vi "FlatToRichni_xnet_can_bm_api_ConnectSettings.vi"(5 "OutputClusterType":T1, 11 "InputCluster":T5) -> (3 "OutputCluster":T1)   [LabVIEW 2025, in "xnet_can_bus_monitor_api_client.lvlib"]
uses:
  ni_xnet_can_bm_api_ConnectSettings_Flat.ctl
  ni_xnet_can_bm_api_CanMode.ctl
  ni_xnet_can_bm_api_Termination.ctl
  ni_xnet_can_bm_api_FdIsoMode.ctl
  ni_xnet_can_bm_api_ConnectSettings.ctl
  xnet_can_bus_monitor_api_client.lvlib
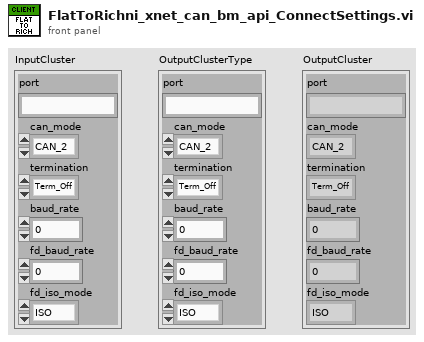
[diagram p1: front panel]
types:
  T1 = typedef "xnet_can_bus_monitor_api_client.lvlib/ni_xnet_can_bm_api_ConnectSettings.ctl" = cluster{"port":string, "can_mode":T2, "termination":T3, "baud_rate":u64, "fd_baud_rate":u64, "fd_iso_mode":T4}
  T2 = typedef "xnet_can_bus_monitor_api_client.lvlib/ni_xnet_can_bm_api_CanMode.ctl" = enum32{"CAN_2", "CAN_FD", "CAN_FD_BRS"}
  T3 = typedef "xnet_can_bus_monitor_api_client.lvlib/ni_xnet_can_bm_api_Termination.ctl" = enum32{"Term_Off", "Term_On"}
  T4 = typedef "xnet_can_bus_monitor_api_client.lvlib/ni_xnet_can_bm_api_FdIsoMode.ctl" = enum32{"ISO", "Non_ISO", "ISO_Legacy"}
  T5 = typedef "xnet_can_bus_monitor_api_client.lvlib/ni_xnet_can_bm_api_ConnectSettings_Flat.ctl" = cluster{"port":string, "can_mode":T2, "termination":T3, "baud_rate":u64, "fd_baud_rate":u64, "fd_iso_mode":T4}
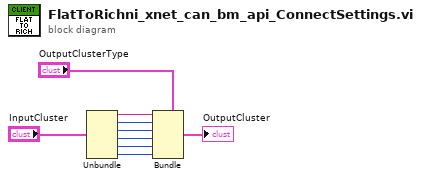
[diagram p0: block diagram]
diagram:
  n1 = Unbundle "Unbundle"("InputCluster") -> ("port"=w6:string, "can_mode"=w5:T2, "termination"=w4:T3, "baud_rate"=w3:u64, "fd_baud_rate"=w2:u64, "fd_iso_mode"=w1:T4)
  n2 = Bundle "Bundle"(cluster="OutputClusterType", "port"=w6, "can_mode"=w5, "termination"=w4, "baud_rate"=w3, "fd_baud_rate"=w2, "fd_iso_mode"=w1) -> (→"OutputCluster":T1)
